vi "WLAN Configure RF.vi"(0 "Instrument Handle In":refnum<k21>, 1 "Selector String":string, 5 "Common Configuration":T1={"Center Frequency (Hz)"=1000000000.0, "Reference Level (dBm)"=0.0, "External Attenuation (dB)"=0.0, "Frequency Reference Source"="OnboardClock", "Digital Edge Source"="PXI_Trig0", "Digital Edge"=0, "Trigger Delay (s)"=0.0, "Enable Trigger?"=TRUE, "LO Source"="LO_In", "LO Offset (Hz)"=0.0} {"External Attenuation (dB)" format="%.2f"; "Reference Level (dBm)" format="%.2f"; "Center Frequency (Hz)" format="%.6p"; "Trigger Delay (s)" format="%.3p"; "Digital Edge" items=["Rising Edge", "Falling Edge"]}, 7 "Auto Level Settings":T2={"Auto Level Reference Level?"=FALSE, "Auto Level Measure Time (s)"=0.01} {"Auto Level Measure Time (s)" format="%#_6p"}, 11 "error in (no error)":errorcluster) -> (4 "Instrument Handle Out":refnum<k21>, 15 "error out":errorcluster)   [LabVIEW 2016, in "RFmxWLAN.lvlib"]
uses:
  RFmxWLAN.lvlib
  Typedefs/WLAN Common Config.ctl
  Typedefs/WLAN AutoLevel Config.ctl
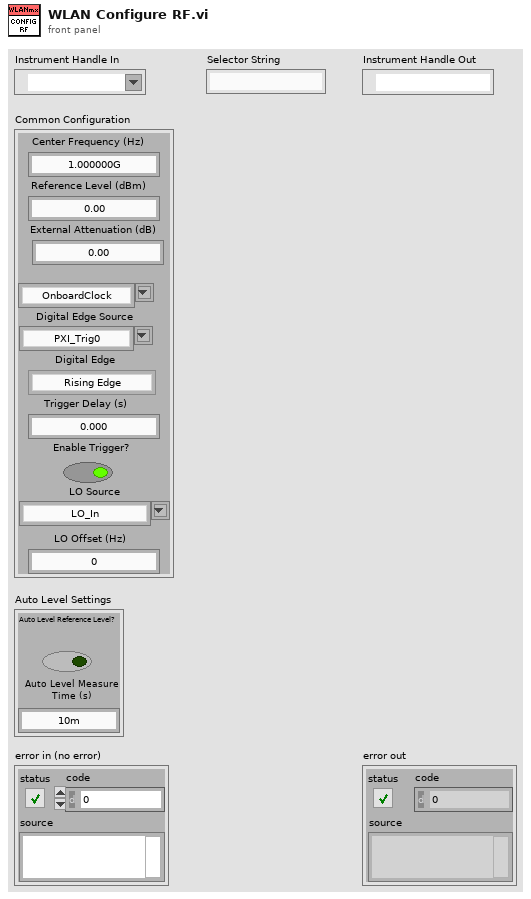
[diagram p1: front panel]
types:
  T1 = typedef "RFmxWLAN.lvlib/WLAN Common Config.ctl" = cluster{"Center Frequency (Hz)":dbl, "Reference Level (dBm)":dbl, "External Attenuation (dB)":dbl, "Frequency Reference Source":string, "Digital Edge Source":string, "Digital Edge":i32, "Trigger Delay (s)":dbl, "Enable Trigger?":bool, "LO Source":string, "LO Offset (Hz)":dbl}
  T2 = typedef "WLAN AutoLevel Config.ctl" = cluster{"Auto Level Reference Level?":bool, "Auto Level Measure Time (s)":dbl}
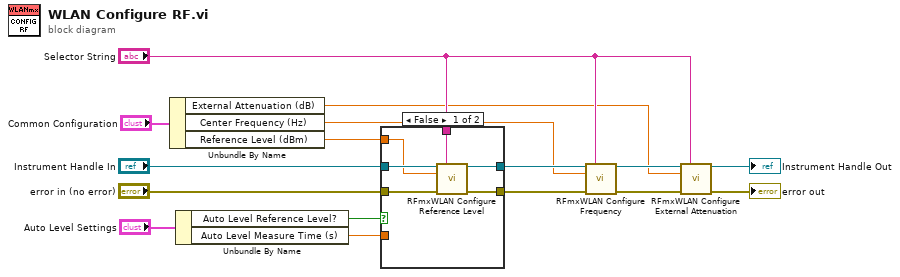
[diagram p0: block diagram]
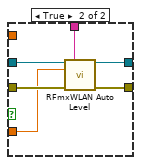
[diagram p2: hidden frame]
diagram:
  n1 = Unbundle By Name("Common Configuration") -> ("External Attenuation (dB)"=w2:dbl, "Center Frequency (Hz)"=w3:dbl, "Reference Level (dBm)"=w4:dbl)
  n2 = Unbundle By Name("Auto Level Settings") -> ("Auto Level Reference Level?"=w6:bool, "Auto Level Measure Time (s)"=w1:dbl)
  n3 = case shown="False" w6 {
    tunnel: "Instrument Handle In" -> [w21 w28]
    tunnel: "Selector String" -> [w18 w27]
    tunnel: "error in (no error)" -> [w22 w26]
    tunnel: [w20 w25] -> w12
    tunnel: [w19 w24] -> w14
    tunnel: w4 -> [w17 _]
    tunnel: w1 -> [_ w23]
    frame False {
      n4 = call <vilib>:"RFmxWLAN Configure Reference Level.vi"("Instrument Handle In"=w21, "Selector String"=w18, "Reference Level"=w17, "error in (no error)"=w22) -> ("Instrument Handle Out"=w20:refnum<k21>, "error out"=w19:errorcluster)  [unwired: 10 in]
    }
    frame True {
      n5 = call <vilib>:"RFmxWLAN Auto Level.vi"("Instrument Handle In"=w28, "Selector String"=w27, "Measurement Interval (s)"=w23, "error in (no error)"=w26) -> ("Instrument Handle Out"=w25:refnum<k21>, "error out"=w24:errorcluster)  [unwired: 10 in]
    }
  }
  n6 = call <vilib>:"RFmxWLAN Configure Frequency.vi"("Instrument Handle In"=w12, "Selector String"="Selector String", "Center Frequency (Hz)"=w3, "error in (no error)"=w14) -> ("Instrument Handle Out"=w10:refnum<k21>, "error out"=w13:errorcluster)  [unwired: 10 in]
  n7 = call <vilib>:"RFmxWLAN Configure External Attenuation.vi"("Instrument Handle In"=w10, "Selector String"="Selector String", "External Attenuation (dB)"=w2, "error in (no error)"=w13) -> ("Instrument Handle Out"=→"Instrument Handle Out":refnum<k21>, "error out"=→"error out":errorcluster)  [unwired: 10 in]
